vi "Push_Data_via_Public_Client.vi"(5 "Archive File?":bool[](array[boolean]), 6 "application reference":refnum<vi>, 7 "error in (no error)":errorcluster, 8 "Running on Server?":bool, 10 "Path of Files relative to EnFlo Data Root":path[](array[path])) -> (0 "error out":errorcluster)   [LabVIEW 2013]
uses:
  Anemometry/Anemometry Sub Vis/Globals/Constants_global.vi
  Sub VIs/Harvest_Global.vi
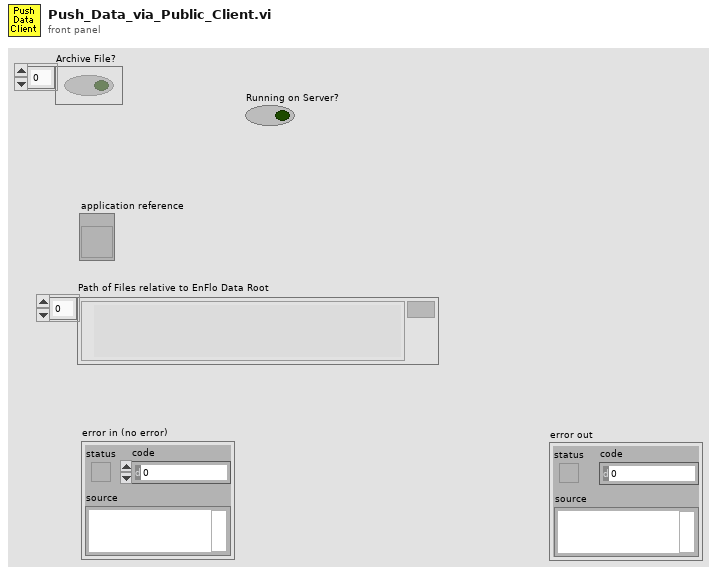
[diagram p1: front panel]
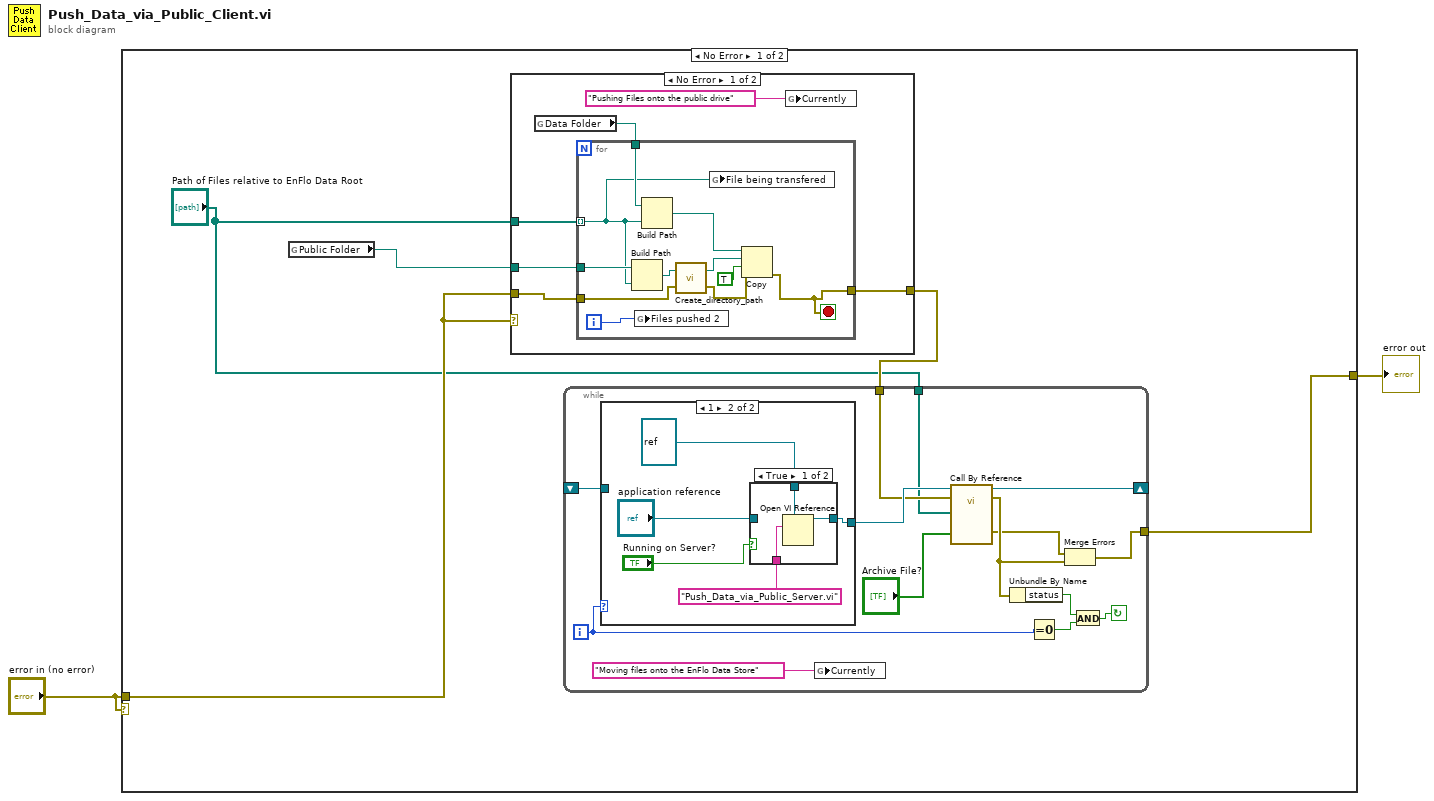
[diagram p0: block diagram]
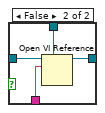
[diagram p3: hidden frame]
diagram:
  n1 = case shown="No Error" "error in (no error)" {
    tunnel: [w5 w53] -> w2
    tunnel: "error in (no error)" -> [w7 w53]
    frame No Error {
      n2 = global read "Constants_global.vi" "Public Folder"() -> (w3:path)
      n3 = case shown="No Error" w7 {
        tunnel: [w36 w52] -> w6
        tunnel: w7 -> [w37 w52]
        tunnel: "Path of Files relative to EnFlo Data Root" -> [w39 _]
        tunnel: w3 -> [w38 _]
        frame No Error {
          n4 = global read "Constants_global.vi" "Data Folder"() -> (w40:path)
          n5 = for {
            tunnel: w40 -> [w43]
            tunnel: w39 -> [w41] mode=indexing
            tunnel: w38 -> [w49]
            tunnel: w37 -> [w45]
            tunnel: [w44] -> w36
            i -> [w42]
            stop <- w44 stop-if-true
            n6 = Build Path(base path=w49, name or relative path=w41) -> (appended path=w50:path)
            n7 = global write "Harvest_Global.vi" "Files pushed 2"(w42) -> ()
            n8 = Build Path(base path=w43, name or relative path=w41) -> (appended path=w51:path)
            n9 = call "Create_directory_path.vi"("error in (no error)"=w45, "Path name"=w50) -> ("error out"=w46:errorcluster, "Path name Out"=w48:path)
            n10 = global write "Harvest_Global.vi" "File being transfered"(w41) -> ()
            n11 = Copy(8:w46, 9:TRUE ("overwrite (F)"), 10:w48, 11:w51) -> (0:w44:errorcluster)  [unwired: 1 in, 2 out]
          }
          n12 = global write "Harvest_Global.vi" "Currently"("Pushing Files onto the public drive" ("Currently Running")) -> ()
        }
        frame Error {
        }
      }
      n13 = while {
        shift-right: [w19] -> _
        shift-left: _ -> [w21]
        tunnel: [w9] -> w5
        tunnel: w6 -> [w13]
        tunnel: "Path of Files relative to EnFlo Data Root" -> [w12]
        i -> [w18]
        stop <- w15 continue-if-true
        n14 = case shown="1" w18 {
          tunnel: w21 -> [w22 _]
          tunnel: [w22 w27] -> w20
          frame 0, Default {
          }
          frame 1 {
            n15 = case shown="True" "Running on Server?" {
              tunnel: [w30 w34] -> w27
              tunnel: "application reference" -> [_ w33]
              tunnel: refnum<vi> refnum ("Push Data Server") -> [w29 w32]
              tunnel: "Push_Data_via_Public_Server.vi" -> [w28 w31]
              frame True {
                n16 = Open VI Reference(type specifier VI Refnum (for type only)=w29, vi path=w28) -> (vi reference=w30:refnum<vi>)  [unwired: 2 in, 3 out]
              }
              frame False {
                n17 = Open VI Reference(type specifier VI Refnum (for type only)=w32, application reference (local)=w33, vi path=w31) -> (vi reference=w34:refnum<vi>)  [unwired: 1 in, 3 out]
              }
            }
          }
        }
        n18 = global write "Harvest_Global.vi" "Currently"("Moving files onto the EnFlo Data Store" ("Currently Running")) -> ()
        n19 = call-by-ref "?"(reference=w20, error in=w13, "Archive File?"="Archive File?", "Path of Files relative to EnFlo Data Root"=w12) -> (reference out=w19:refnum<vi>, error out=w11:errorcluster, "error out"=w10:errorcluster)  [unwired: 2 in]
        n20 = Unbundle By Name(w11) -> ("status"=w16:bool)
        n21 = Equal To 0?(x=w18) -> (x = 0?=w17:bool)
        n22 = Merge Errors(w10, w11) -> (w9:errorcluster)
        n23 = And(x=w16, y=w17) -> (x .and. y?=w15:bool)
      }
    }
    frame Error {
    }
  }
  "error out" <- w2
